vi "Error_ToSpecificClass.vi"(8 "error in (no error)":errorcluster, 10 "Control Label":string) -> (0 "error out":errorcluster)   [LabVIEW 2020, in "CtlReferences.lvlib" / "CtlReferences.lvclass"]
doc: "This VI will insert the error if an incorrect class conversion is attempted on a reference"
uses:
  CtlReferences.lvclass
  CtlReferences.lvclass/CtlReferences.ctl
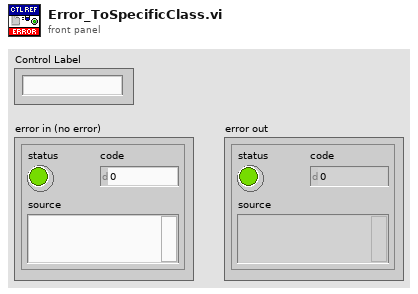
[diagram p1: front panel]
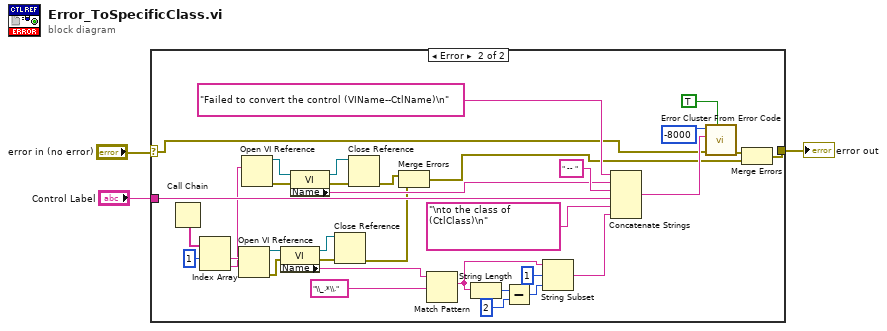
[diagram p0: block diagram]
diagram:
  n1 = case shown="Error" "error in (no error)" {
    selector: "error in (no error)" -> [w4 w13]
    tunnel: [w4 w6] -> w2
    tunnel: "Control Label" -> [_ w26]
    frame No Error {
    }
    frame Error {
      n2 = Call Chain() -> (call chain=w20:string[])
      n3 = Index Array(array=w20, index #1=1 ("index")) -> (element #1=w21:string, element #2=w17:string)  [unwired: 1 in]
      n4 = Open VI Reference(vi path=w21) -> (vi reference=w18:refnum<vi>, error out=w9:errorcluster)  [unwired: 5 in]
      n5 = Open VI Reference(vi path=w17) -> (vi reference=w16:refnum<vi>, error out=w12:errorcluster)  [unwired: 5 in]
      n6 = property class="VI"(reference=w18, error in=w9) -> (reference out=w10:refnum<vi>, error out=w11:errorcluster, "Name"=w33:string)
      n7 = property class="VI"(reference=w16, error in=w12) -> (reference out=w14:refnum<vi>, error out=w15:errorcluster, "Name"=w36:string)
      n8 = Close Reference(reference=w10, error in (no error)=w11) -> (error out=w7:errorcluster)
      n9 = Close Reference(reference=w14, error in (no error)=w15) -> (error out=w8:errorcluster)
      n10 = Merge Errors(w8, w7) -> (w5:errorcluster)
      n11 = Match Pattern(string=w33, regular expression="\\_.*\\.") -> (match substring=w28:string)  [unwired: 1 in, 3 out]
      n12 = String Length(string=w28) -> (length=w30:i32)
      n13 = Subtract(x=w30, y=2) -> (x-y=w31:i32)
      n14 = String Subset(string=w28, offset (0)=1, length (rest)=w31) -> (substring=w27:string)
      n15 = Concatenate Strings("Failed to convert the control (VIName--CtlName)\n" ("source"), w36, " -- " ("string"), w26, "\nto the class of (CtlClass)\n" ("source"), w27) -> (w24:string)
      n16 = call <vilib>:"Error Cluster From Error Code.vi"("show call chain? (False)"=TRUE, "error in (no error)"=w13, "error message (\"\")"=w24, "error code (0)"=-8000 ("NewError code")) -> ("error out"=w25:errorcluster)  [unwired: 5 in]
      n17 = Merge Errors(w25, w5) -> (w6:errorcluster)
    }
  }
  "error out" <- w2
